vi "题目6.1.vi"   [LabVIEW 2017]
types:
  T1 = enum16{"open", "replace", "create", "open or create", "replace or create", "replace or create with confirmation"}
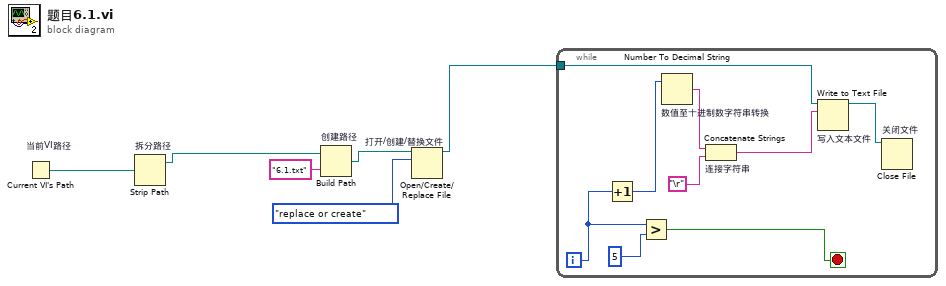
[diagram p0: block diagram]
diagram:
  n1 = Current VI's Path "当前VI路径"() -> (path=w2:path)
  n2 = Strip Path "拆分路径"(path=w2) -> (stripped path=w3:path)  [unwired: 1 out]
  n3 = Build Path "创建路径"(base path=w3, name or relative path="6.1.txt" ("名称或相对路径")) -> (appended path=w5:path)
  n4 = Open/Create/Replace File "打开/创建/替换文件"(file path (use dialog)=w5, operation (0:open)=T1."replace or create" ("操作(0:open)")) -> (refnum out=w1:refnum<file>)  [unwired: 4 in, 2 out]
  n5 = while {
    tunnel: w1 -> [w7]
    i -> [w15]
    stop <- w13 stop-if-true
    n6 = Increment(x=w15) -> (x+1=w12:i32)
    n7 = Greater?(x=w15, y=5) -> (0:w13:bool)
    n8 = Number To Decimal String "数值至十进制数字符串转换"(number=w12) -> (decimal integer string=w11:string)  [unwired: 1 in]
    n9 = Concatenate Strings "连接字符串"(w11, "\r") -> (w9:string)
    n10 = Write to Text File "写入文本文件"(file (use dialog)=w7, text=w9) -> (refnum out=w8:refnum<file>)  [unwired: 2 in, 2 out]
    n11 = Close File "关闭文件"(refnum=w8) -> ()  [unwired: 1 in, 2 out]
  }
